vi "parola sorgu programı.vi"() -> ()   [LabVIEW 2014]
panel:
  out "?":bool
  out "doğruluk":string
  in  "şifre":dbl
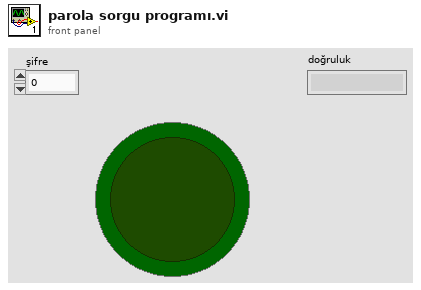
[diagram p1: front panel]
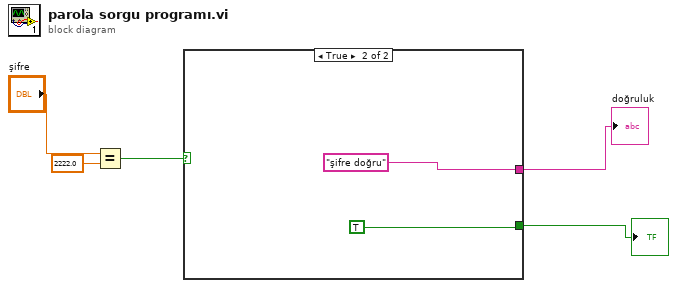
[diagram p0: block diagram]
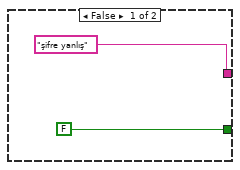
[diagram p2: hidden frame]
diagram:
  n1 = Equal?(x="şifre", y=2222.0) -> (x = y?=w1:bool)
  n2 = case shown="True" w1 {
    tunnel: ["şifre yanlış" "şifre doğru"] -> w3
    tunnel: [FALSE TRUE] -> w2
    frame False {
    }
    frame True {
    }
  }
  "doğruluk" <- w3
  "?" <- w2
